vi "Read Owning System.vi"(8 "error in (no error)":errorcluster, 11 "Generic Hardware in":refnum<class "Generic Hardware.lvclass">) -> (0 "error out":errorcluster, 2 "Owning System":T1, 3 "Generic Hardware out":refnum<class "Generic Hardware.lvclass">)   [LabVIEW 2017, in "Generic Hardware.lvclass"]
uses:
  Generic Hardware.lvclass
  Type Defs/Owning System.ctl
  Generic Hardware.lvclass/Generic Hardware.ctl
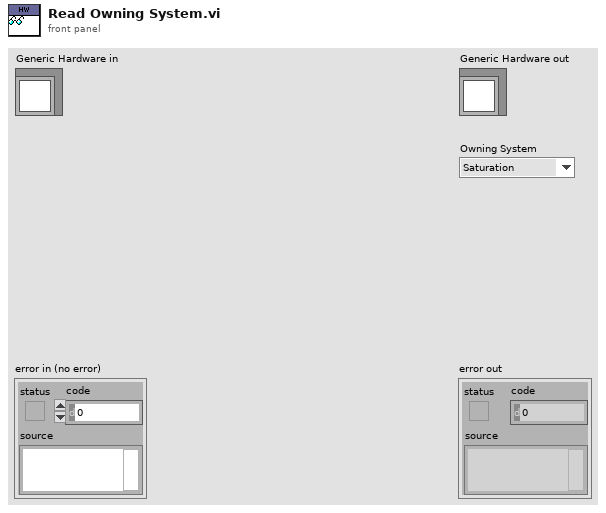
[diagram p1: front panel]
types:
  T1 = typedef "Generic Hardware.lvclass/Owning System.ctl" = enum16{"Saturation", "Expansion"}
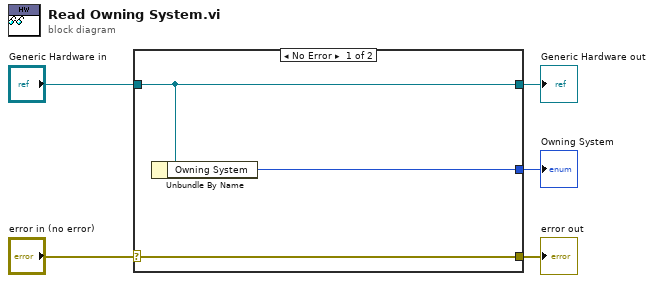
[diagram p0: block diagram]
diagram:
  n1 = case shown="No Error" "error in (no error)" {
    selector: "error in (no error)" -> [w8 w9]
    tunnel: [w8 w9] -> w4
    tunnel: [w7 w10] -> w2
    tunnel: "Generic Hardware in" -> [w7 w10]
    tunnel: [w6 _] -> w1
    frame No Error {
      n2 = Unbundle By Name(w7) -> ("Owning System"=w6:T1)
    }
    frame Error {
    }
  }
  "error out" <- w4
  "Generic Hardware out" <- w2
  "Owning System" <- w1
